vi "Team # to IP Address.vi"(7 "Update":bool, 10 "Team #":u32) -> (2 "Team IP Address":string)   [LabVIEW 2025]
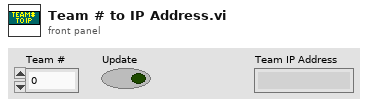
[diagram p1: front panel]
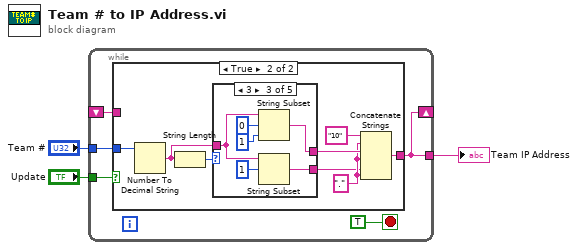
[diagram p0: block diagram]
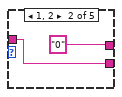
[diagram p4: hidden frame]
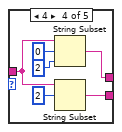
[diagram p5: hidden frame]
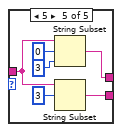
[diagram p6: hidden frame]
diagram:
  n1 = while {
    tunnel: "Team #" -> [w8]
    tunnel: [w7] -> w2
    shift-right: [w7] -> _
    shift-left: _ -> [w4]
    tunnel: "Update" -> [w5]
    stop <- TRUE stop-if-true
    n2 = case shown="True" w5 {
      tunnel: w8 -> [_ w17]
      tunnel: [w9 w10] -> w7
      tunnel: w4 -> [w9 _]
      frame False {
      }
      frame True {
        w13 = "." ("string")
        n3 = Number To Decimal String(number=w17) -> (decimal integer string=w11:string)  [unwired: 1 in]
        n4 = String Length(string=w11) -> (length=w15:i32)
        n5 = case shown="3" w15 {
          tunnel: w11 -> [_ w19 w23 w29 w35]
          tunnel: [_ "0" w21 w27 w33] -> w14
          tunnel: [_ w19 w25 w31 w37] -> w12
          frame 0, Default {
          }
          frame 1, 2 {
          }
          frame 3 {
            n6 = String Subset(string=w23, offset (0)=0, length (rest)=1 ("length (rest)")) -> (substring=w21:string)
            n7 = String Subset(string=w23, offset (0)=1) -> (substring=w25:string)  [unwired: 1 in]
          }
          frame 4 {
            n8 = String Subset(string=w29, offset (0)=0, length (rest)=2 ("length (rest)")) -> (substring=w27:string)
            n9 = String Subset(string=w29, offset (0)=2) -> (substring=w31:string)  [unwired: 1 in]
          }
          frame 5 {
            n10 = String Subset(string=w35, offset (0)=0, length (rest)=3 ("length (rest)")) -> (substring=w33:string)
            n11 = String Subset(string=w35, offset (0)=3) -> (substring=w37:string)  [unwired: 1 in]
          }
        }
        n12 = Concatenate Strings("10" ("string"), w13, w14, w13, w12, w13) -> (w10:string)
      }
    }
  }
  "Team IP Address" <- w2
